vi "comp_stop2.vi"(0 "VISA resource name":refnum<visa-resource-name>, 5 "Master Axis":i32, 7 "Slave Axis":i32, 9 "Reduction Ratio (0)":dbl=1.0, 11 "error in (no error)":errorcluster, 12 "Velocity (units/s)":dbl min=0.0 format="%.4g", 13 "Acceleration (0 units/s²)":dbl min=0.0 format="%.4g") -> (4 "VISA resource name out":refnum<visa-resource-name>, 15 "error out":errorcluster)   [LabVIEW 2011]
uses:
  <instrlib>/Newport ESP301/Newport ESP301.lvlib
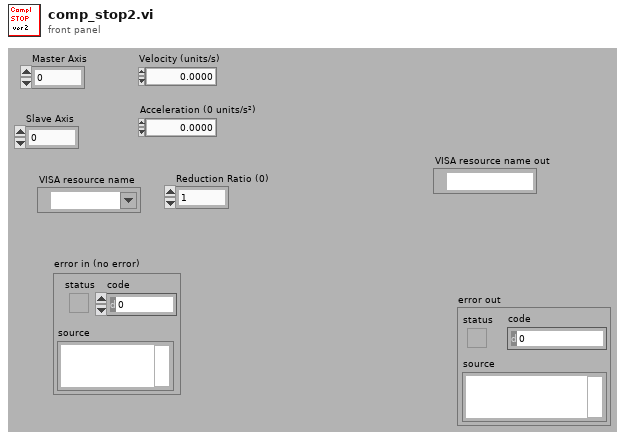
[diagram p1: front panel]
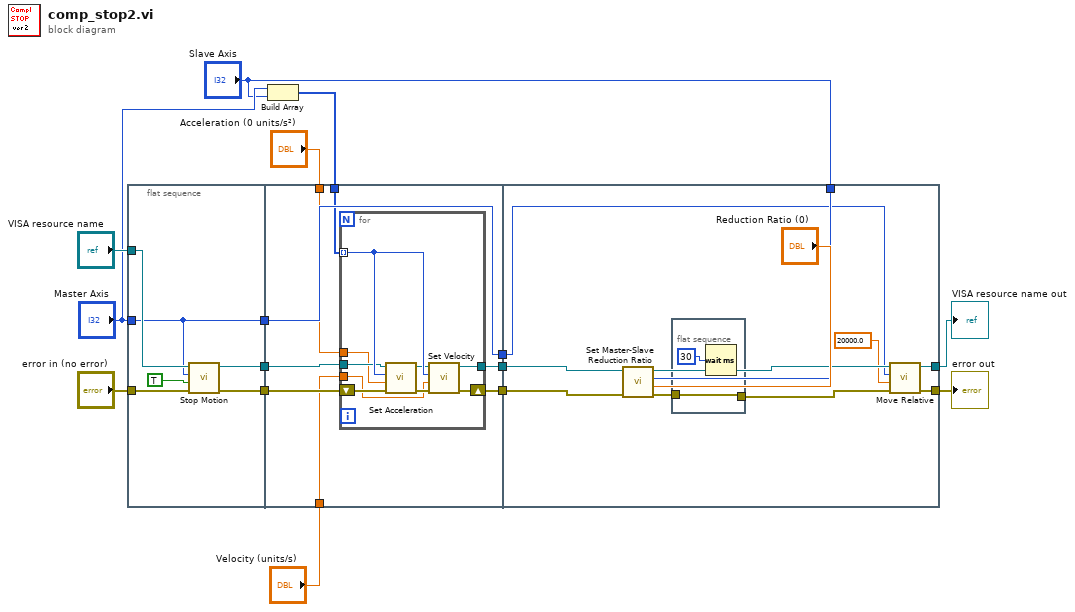
[diagram p0: block diagram]
diagram:
  n1 = flat-sequence {
    tunnel: "VISA resource name" -> [w20]
    tunnel: "Master Axis" -> [w16]
    tunnel: "error in (no error)" -> [w19]
    tunnel: [w18] -> w11
    tunnel: [w17] -> w9
    tunnel: [w16] -> w7
    tunnel: w11 -> [w25]
    tunnel: [w22] -> w10
    tunnel: w9 -> [w27]
    tunnel: [w26] -> w8
    tunnel: w7 -> [w29]
    tunnel: [w29] -> w6
    tunnel: w4 -> [w28]
    tunnel: "Acceleration (0 units/s²)" -> [w24]
    tunnel: "Velocity (units/s)" -> [w23]
    tunnel: w10 -> [w41]
    tunnel: w8 -> [w42]
    tunnel: w6 -> [w43]
    tunnel: "Slave Axis" -> [w44]
    tunnel: [w46] -> w13
    tunnel: [w45] -> w12
    frame #0 {
      n2 = call <instrlib>:"Stop Motion.vi"("error in (no error)"=w19, "Stop all axes (F)"=TRUE, "Axis (1)"=w16, "VISA resource name"=w20) -> ("error out"=w18:errorcluster, "VISA resource name out"=w17:refnum<visa-resource-name>)  [unwired: 2 in]
    }
    frame #1 {
      n3 = for {
        tunnel: w28 -> [w38] mode=indexing
        tunnel: w27 -> [w37]
        tunnel: [w35] -> w26
        tunnel: w24 -> [w31]
        tunnel: w23 -> [w30]
        shift-right: [w32] -> w22
        shift-left: w25 -> [w34]
        n4 = call <instrlib>:"Set Acceleration.vi"("error in (no error)"=w34, "Acceleration (0 units/s²)"=w31, "Axis (1)"=w38, "VISA resource name"=w37) -> ("error out"=w33:errorcluster, "VISA resource name out"=w36:refnum<visa-resource-name>)  [unwired: 2 in]
        n5 = call <instrlib>:"Set Velocity.vi"("error in (no error)"=w33, "Velocity (units/s)"=w30, "Axis (1)"=w38, "VISA resource name"=w36) -> ("error out"=w32:errorcluster, "VISA resource name out"=w35:refnum<visa-resource-name>)  [unwired: 2 in]
      }
    }
    frame #2 {
      n6 = call <instrlib>:"Set Master-Slave Reduction Ratio.vi"("error in (no error)"=w41, "Reduction Ratio (0)"="Reduction Ratio (0)", "Axis (1)"=w44, "VISA resource name"=w42) -> ("error out"=w40:errorcluster, "VISA resource name out"=w48:refnum<visa-resource-name>)  [unwired: 2 in]
      n7 = flat-sequence {
        tunnel: [w51] -> w39
        tunnel: w40 -> [w51]
        frame #0 {
          n8 = Wait (ms)(milliseconds to wait=u32 30) -> ()  [unwired: 1 out]
        }
      }
      n9 = call <instrlib>:"Move Relative.vi"("error in (no error)"=w39, "Position (0 units)"=20000.0, "Axis (1)"=w43, "VISA resource name"=w48) -> ("error out"=w46:errorcluster, "VISA resource name out"=w45:refnum<visa-resource-name>)  [unwired: 2 in]
    }
  }
  n10 = Build Array("Master Axis", "Slave Axis") -> (w4:i32[])
  "error out" <- w13
  "VISA resource name out" <- w12
